vi "VI-File-Explorer.vi"() -> ()   [LabVIEW 2011, in "vi_lib.lvlib"]
uses:
  vi_lib.lvlib
  clLabview/clLabview.lvclass
  clFile/clFile.lvclass
panel:
  out "VI Name":string
  in  "new VI-Lib Password":string
  in  "Update LV-Lib Password":bool
  out "File is protected?":bool=TRUE
  out "LV-Lib password (Hex)":string
  out "Icon":picture
  out "busy (*)":bool
  out "Salt (Hex)":string
  out "MD5-Hash 2 (Hex)":string
  out "MD5-Hash 1 (Hex)":string
  out "saving done":bool
  in  "save":bool
  in  "Open":bool
  in  "stop":bool
  out "flags":i32 step=1
  out "stage":u8(ring) items=["development", "alpha", "beta", "release"]
  out "build":u8 step=1
  out "bugfix":u8 step=1
  out "minor":u8 max=99 step=1
  out "major":u8=3 min=1 max=99 step=1
  out "version info":string
  out "version text":string
  out "save to":path=path "D:/labview/file_in_(free).vi"
  in  "new File Password":string
  in  "open from":path=path "D:/labview/file.vi"
  out "MD5 password (Hex)":string
  # "File password [BDPW]"
  # "Open"
  # "for LV-Version >= 8"
  # "for LV-Version >= 12"
  # "Save"
  # "File propertys [LVSR]"
  # "File version [vers]"
  # "(*) This is a \"brute force\" version to calc the password Salt, \n      so it might take up to 30sec."
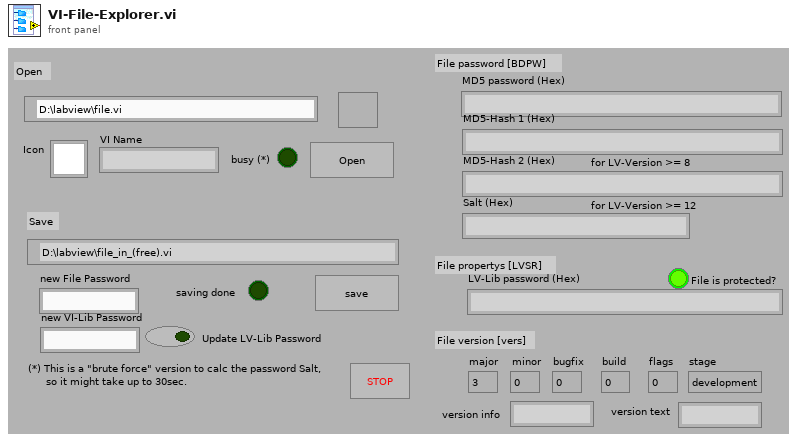
[diagram p1: front panel]
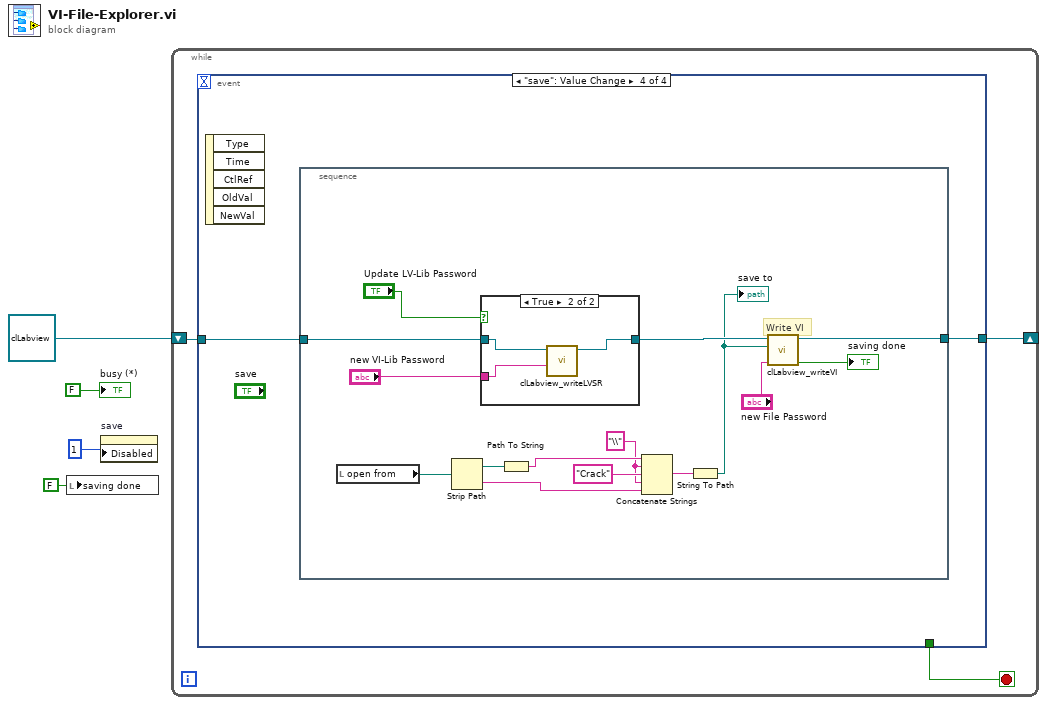
[diagram p0: block diagram]
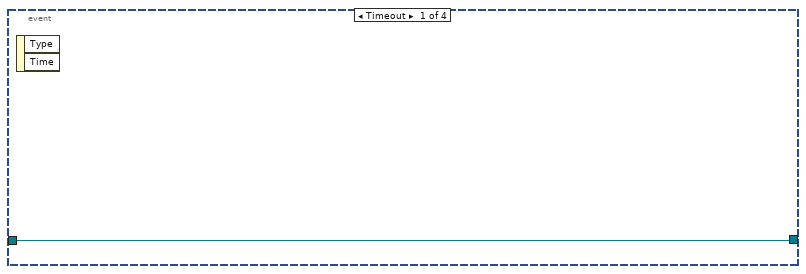
[diagram p2: hidden frame]
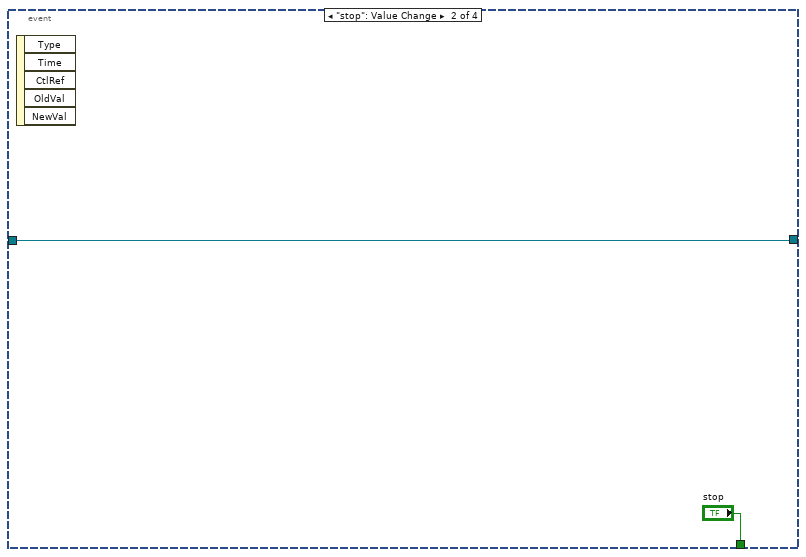
[diagram p3: hidden frame]
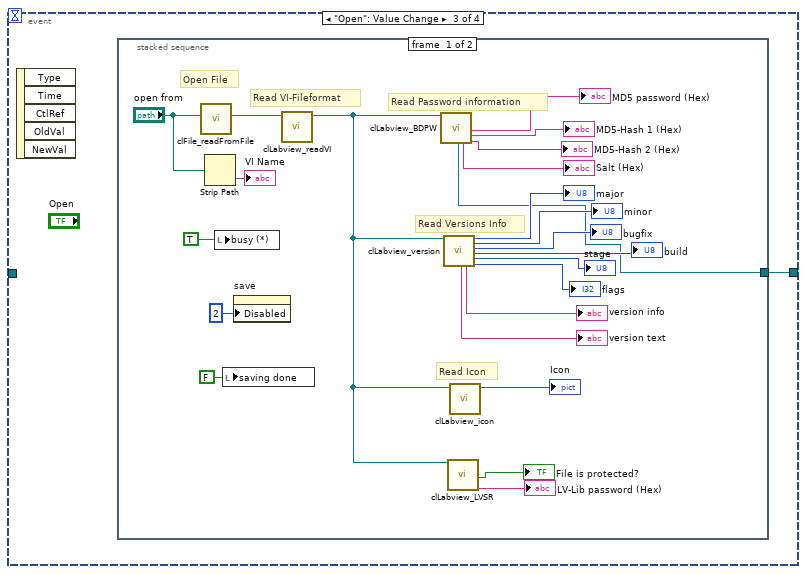
[diagram p4: hidden frame]
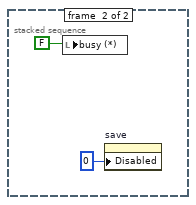
[diagram p5: hidden frame]
diagram:
  n1 = local write "saving done"(FALSE ("saving done")) -> ()
  n2 = property on="save" class="Bool"("Disabled"=u8 1) -> ()  [unwired: 2 in, 2 out]
  n3 = while {
    shift-right: [w5] -> _
    shift-left: refnum<class "clLabview.lvclass"> refnum ("vi_lib.lvlib:clLabview.lvclass 2") -> [w6]
    stop <- w7 stop-if-true
    n4 = event shown="[3] \"save\": Value Change" {
      selector: _ -> [_ _ _ _]
      dyn-events: _ -> [_ _ _ _]
      timeout: _ -> [_ _ _ _]
      tunnel: [_ "stop" _ _] -> w7
      tunnel: w6 -> [w8 w9 _ w38]
      tunnel: [w8 w9 w11 w37] -> w5
      event Timeout {
        n5 = event-data() -> ()  [unwired: 1 in, 2 out]
      }
      event "stop": Value Change {
        n6 = event-data() -> ()  [unwired: 1 in, 5 out]
      }
      event "Open": Value Change {
        n7 = event-data() -> ()  [unwired: 1 in, 5 out]
        n8 = stacked-sequence {
          tunnel: [w15 _] -> w11
          frame #0 {
            # "Read Icon"
            # "Read Versions Info"
            # "Read Password information"
            # "Read VI-Fileformat"
            # "Open File"
            n9 = call "clFile_readFromFile.vi"("file (use dialog)"="open from") -> ("clFileReader.lvclass"=w19:refnum<class "clFileReader.lvclass">)  [unwired: 1 in, 9 out]
            n10 = Strip Path(path="open from") -> (name=→"VI Name":string)  [unwired: 1 out]
            n11 = local write "busy (*)"(TRUE ("busy")) -> ()
            n12 = local write "saving done"(FALSE ("saving done")) -> ()
            n13 = property on="save" class="Bool"("Disabled"=u8 2) -> ()  [unwired: 2 in, 2 out]
            n14 = call "clLabview_readVI.vi"("vi_lib.lvlib:clFileReader.lvclass"=w19) -> ("vi_lib.lvlib:clLabview.lvclass 2"=w32:refnum<class "clLabview.lvclass">)  [unwired: 10 out]
            n15 = call "clLabview_BDPW.vi"("vi_lib.lvlib:clLabview.lvclass"=w32) -> ("vi_lib.lvlib:clLabview.lvclass [Out]"=w15:refnum<class "clLabview.lvclass">, "Salt (Hex)"=→"Salt (Hex)":string, "MD5 password (Hex)"=→"MD5 password (Hex)":string, "MD5-Hash 1  (Hex)"=→"MD5-Hash 1 (Hex)":string, "MD5-Hash 2  (Hex)"=→"MD5-Hash 2 (Hex)":string)  [unwired: 14 out]
            n16 = call "clLabview_version.vi"("vi_lib.lvlib:clLabview.lvclass"=w32) -> ("version_text"=→"version text":string, "version_info"=→"version info":string, "major"=→"major":u8, "minor"=→"minor":u8, "bugfix"=→"bugfix":u8, "build"=→"build":u8, "stage"=→"stage":u8, "flags"=→"flags":i32)  [unwired: 11 out]
            n17 = call "clLabview_LVSR.vi"("vi_lib.lvlib:clLabview.lvclass"=w32) -> ("File is protected?"=→"File is protected?":bool, "MD5 lib Password (Hex)"=→"LV-Lib password (Hex)":string)  [unwired: 17 out]
            n18 = call "clLabview_icon.vi"("vi_lib.lvlib:clLabview.lvclass"=w32) -> ("Icon"=→"Icon":picture)  [unwired: 10 out]
          }
          frame #1 {
            n19 = local write "busy (*)"(FALSE ("busy")) -> ()
            n20 = property on="save" class="Bool"("Disabled"=u8 0) -> ()  [unwired: 2 in, 2 out]
          }
        }
      }
      event "save": Value Change {
        n21 = event-data() -> ()  [unwired: 1 in, 5 out]
        n22 = stacked-sequence {
          tunnel: w38 -> [w47]
          tunnel: [w46] -> w37
          frame #0 {
            w40 = "\\"
            # "Write VI"
            n23 = local read "open from"() -> (w53:path)
            n24 = Strip Path(path=w53) -> (stripped path=w45:path, name=w39:string)
            n25 = case shown="True" "Update LV-Lib Password" {
              tunnel: w47 -> [w54 w57]
              tunnel: [w54 w56] -> w50
              tunnel: "new VI-Lib Password" -> [_ w55]
              frame False {
              }
              frame True {
                n26 = call "clLabview_writeLVSR.vi"("vi_lib.lvlib:clLabview.lvclass"=w57, "new lib Password"=w55) -> ("vi_lib.lvlib:clLabview.lvclass [Out]"=w56:refnum<class "clLabview.lvclass">)  [unwired: 8 out]
              }
            }
            n27 = Path To String(path=w45) -> (string=w44:string)
            n28 = Concatenate Strings(w44, w40, "Crack" ("string"), w40, w39) -> (w42:string)
            n29 = String To Path(string=w42) -> (path=w41:path)
            "save to" <- w41
            n30 = call "clLabview_writeVI.vi"("vi_lib.lvlib:clLabview.lvclass"=w50, "filename (use dialog)"=w41, "new Password"="new File Password") -> ("vi_lib.lvlib:clLabview.lvclass [Out]"=w46:refnum<class "clLabview.lvclass">, "no Error"=→"saving done":bool)  [unwired: 6 out]
          }
        }
      }
    }
  }
  "busy (*)" <- FALSE ("busy")
